vi "UpperCase (1).vi"() -> ()   [LabVIEW 2015]
panel:
  in  "stop":bool
  in  "String":string
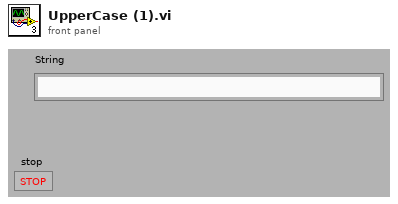
[diagram p1: front panel]
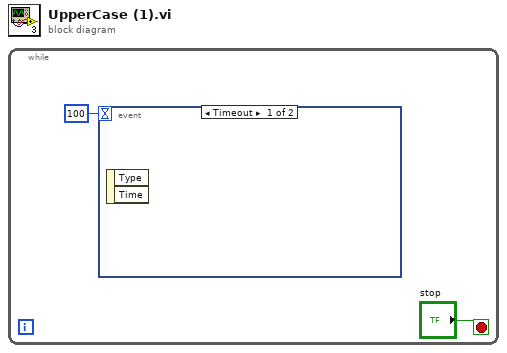
[diagram p0: block diagram]
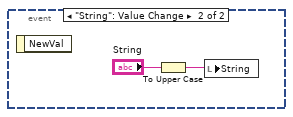
[diagram p2: hidden frame]
diagram:
  n1 = while {
    stop <- "stop" stop-if-true
    n2 = event shown="[0] Timeout" {
      selector: _ -> [_ _]
      dyn-events: _ -> [_ _]
      timeout: 100 -> [_ _]
      event Timeout {
        n3 = event-data() -> ()  [unwired: 1 in, 2 out]
      }
      event "String": Value Change {
        n4 = event-data() -> ()  [unwired: 1 in, 1 out]
        n5 = To Upper Case(1:"String") -> (0:w3:string)
        n6 = local write "String"(w3) -> ()
      }
    }
  }
